vi "ex_ParseFileHeader.vi"(8 "error in (no error)":errorcluster, 11 "file header string":string) -> (0 "error out":errorcluster, 1 "Timestamp":timestamp format="%<%X\n%x>T", 2 "delimiter":string, 3 "file_params":T2={"include col headings?"=TRUE, "x_columns"=0, "col headings always?"=TRUE, "time preference"=0, "hide col headings"=FALSE} {"time preference" items=["Absolute", "Relative"]; "x_columns" items=["None", "One", "Multiple"]}, 4 "optional info":T1, 5 "Decimal Separator":string)   [LabVIEW 2017]
uses:
  <vilib>/express/express input/ExFileReadBlock.llb/ex_ReadFileParams.ctl
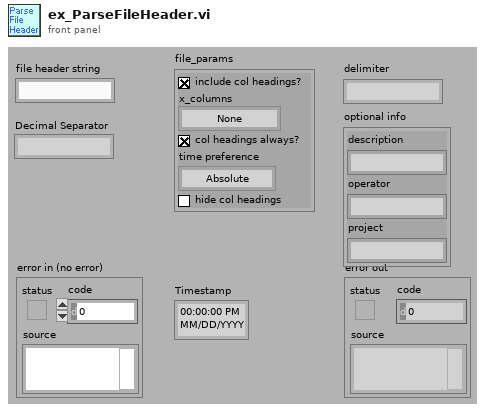
[diagram p1: front panel]
types:
  T1 = cluster{"description":string, "operator":string, "project":string}
  T2 = typedef "ex_ReadFileParams.ctl" = cluster{"include col headings?":bool, "x_columns":u16, "col headings always?":bool, "time preference":u16, "hide col headings":bool}
  T3 = cluster{"Date?":bool, "Time?":bool, "WriterVer?":bool, "ReaderVer?":bool}
  T4 = cluster{"Date":string, "Time":string, "WriterVer":string, "ReaderVer":string}
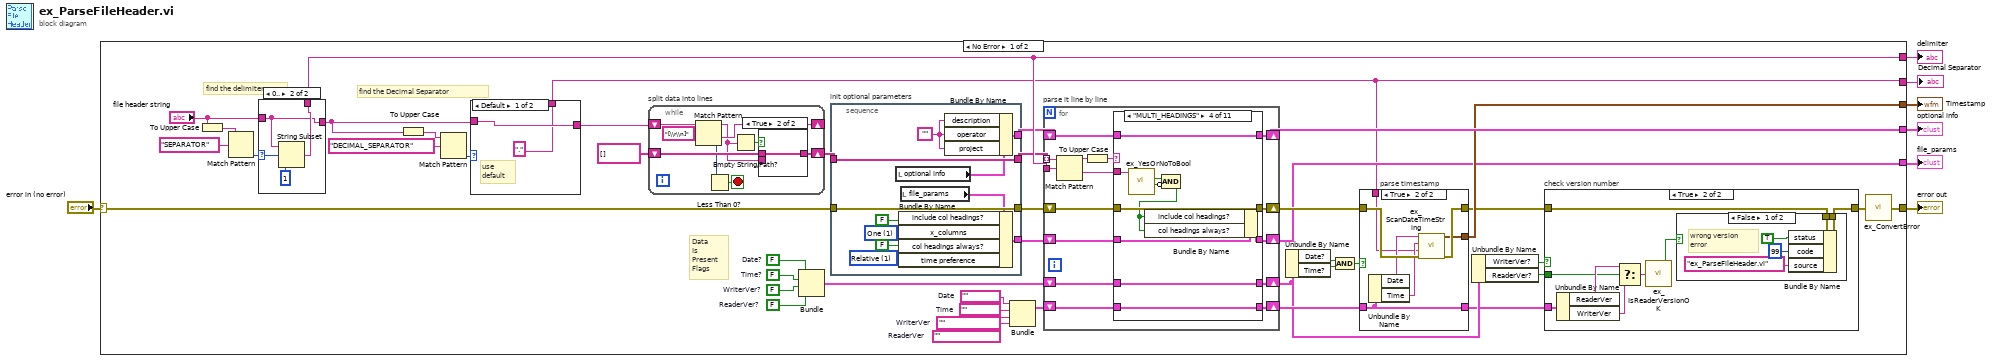
[diagram p0: block diagram]
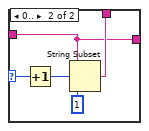
[diagram p2: hidden frame]
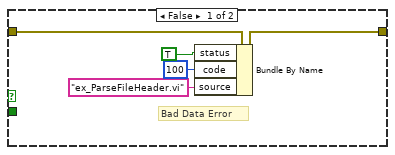
[diagram p3: hidden frame]
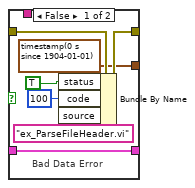
[diagram p5: hidden frame]
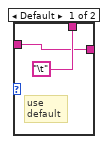
[diagram p6: hidden frame]
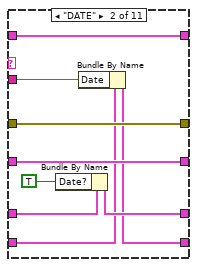
[diagram p8: hidden frame]
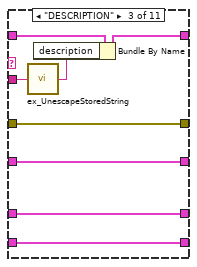
[diagram p9: hidden frame]
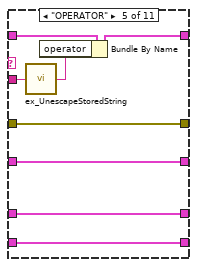
[diagram p10: hidden frame]
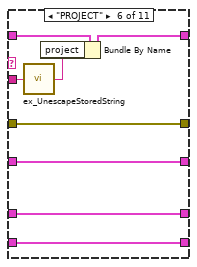
[diagram p11: hidden frame]
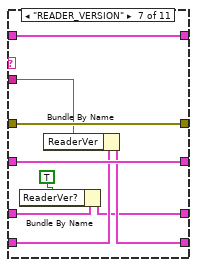
[diagram p12: hidden frame]
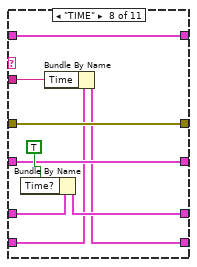
[diagram p13: hidden frame]
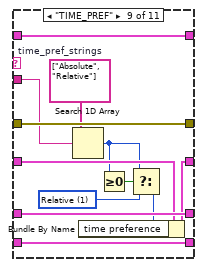
[diagram p14: hidden frame]
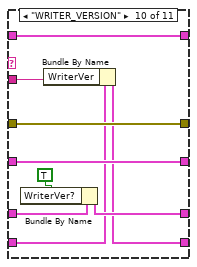
[diagram p15: hidden frame]
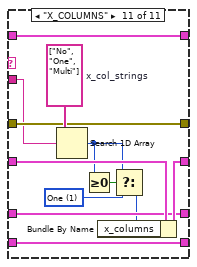
[diagram p16: hidden frame]
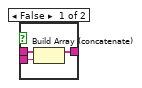
[diagram p17: hidden frame]
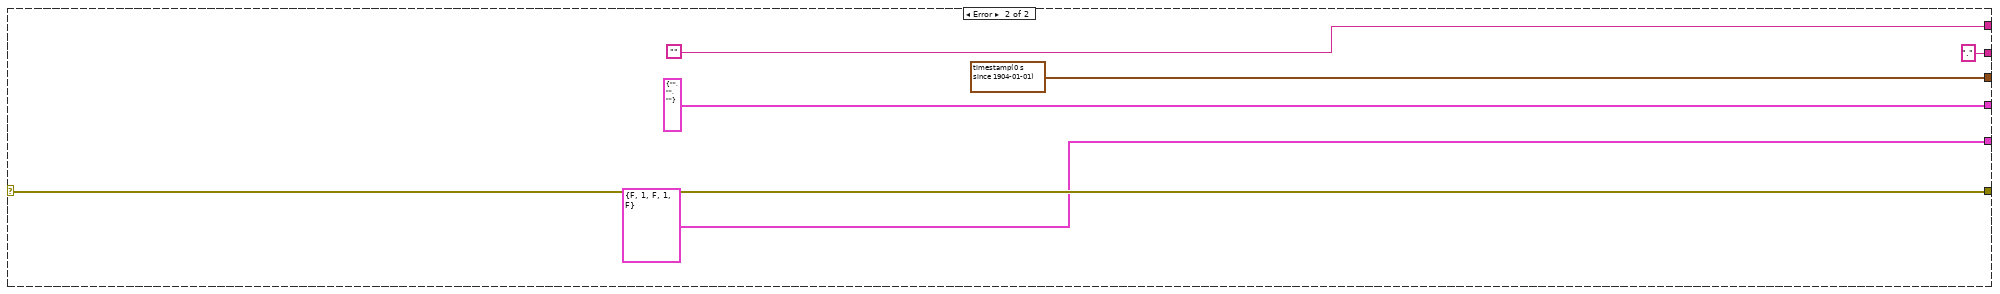
[diagram p18: hidden frame]
diagram:
  n1 = case shown="No Error" "error in (no error)" {
    selector: "error in (no error)" -> [w38 w240]
    tunnel: [w16 w240] -> w6
    tunnel: [w49 ""] -> w5
    tunnel: [w35 T1 {"description"="", "operator"="", "project"=""} ("optional info")] -> w3
    tunnel: [w17 T2 {"include col headings?"=FALSE, "x_columns"=1, "col headings always?"=FALSE, "time preference"=1, "hide col headings"=FALSE} ("file_params")] -> w4
    tunnel: [w23 timestamp(0 s since 1904-01-01)] -> w2
    tunnel: [w8 "." ("file header string")] -> w1
    frame No Error {
      w31 = ""  # ReaderVer
      w30 = ""  # WriterVer
      w32 = FALSE  # ReaderVer?
      w29 = ""  # Time
      w34 = ""  # Date
      w43 = FALSE  # WriterVer?
      w45 = FALSE  # Time?
      w44 = FALSE  # Date?
      # "find the Decimal Separator"
      # "Data\nIs\nPresent\nFlags"
      # "find the delimiter"
      n2 = To Upper Case(1:"file header string") -> (0:w12:string)
      n3 = Match Pattern(string=w12, regular expression="SEPARATOR") -> (offset past match=w47:i32)  [unwired: 4 out]
      n4 = case shown="0.." w47 {
        selector: w47 -> [_ w105]
        tunnel: "file header string" -> [w102 w104]
        tunnel: ["\t" w107] -> w49
        tunnel: [w102 w104] -> w10
        frame Default {
          # "use\ndefault"
        }
        frame 0.. {
          n5 = String Subset(string=w104, offset (0)=w105, length (rest)=1 ("length (rest)")) -> (substring=w107:string)
        }
      }
      n6 = To Upper Case(1:w10) -> (0:w9:string)
      n7 = Match Pattern(string=w9, regular expression="DECIMAL_SEPARATOR") -> (offset past match=w13:i32)  [unwired: 4 out]
      n8 = case shown="Default" w13 {
        selector: w13 -> [_ w54]
        tunnel: w10 -> [w52 w55]
        tunnel: ["." w57] -> w8
        tunnel: [w52 w55] -> w11
        frame Default {
          # "use\ndefault"
        }
        frame 0.. {
          n9 = Increment(x=w54) -> (x+1=w53:i32)
          n10 = String Subset(string=w55, offset (0)=w53, length (rest)=1 ("length (rest)")) -> (substring=w57:string)
        }
      }
      n11 = while "split data into lines" {
        shift-right: [w224] -> _
        shift-left: w11 -> [w230]
        shift-right: [w228] -> w41
        shift-left: string[] [] -> [w229]
        stop <- w226 stop-if-true
        n12 = Match Pattern(string=w230, regular expression="[\\r\\n]") -> (before substring=w223:string, after substring=w224:string, offset past match=w227:i32)  [unwired: 2 out]
        n13 = Less Than 0?(x=w227) -> (x < 0?=w226:bool)
        n14 = Empty String/Path?(string/path=w223) -> (empty?=w222:bool)
        n15 = case shown="True" w222 {
          tunnel: w229 -> [w233 w234]
          tunnel: w223 -> [w232 _]
          tunnel: [w231 w234] -> w228
          frame False {
            n16 = Build Array (concatenate)(w233, w232) -> (w231:string[])
          }
          frame True {
          }
        }
      }
      n17 = Bundle("Date?"=w44, "Time?"=w45, "WriterVer?"=w43, "ReaderVer?"=w32) -> (w42:T3)  [unwired: 1 out]
      n18 = stacked-sequence "init optional parameters" {
        tunnel: w41 -> [w101]
        tunnel: [w101] -> w40
        tunnel: [w100] -> w39
        tunnel: w38 -> [w100]
        tunnel: [w94] -> w37
        tunnel: [w92] -> w36
        frame #0 {
          w91 = ""
          w95 = u16 1 items=["Absolute", "Relative"] ("time preference")
          w97 = u16 1 items=["None", "One", "Multiple"] ("x_columns")
          n19 = local read "optional info"() -> (w93:T1)
          n20 = local read "file_params"() -> (w99:T2)
          n21 = Bundle By Name(cluster=w99, "include col headings?"=FALSE, "x_columns"=w97, "col headings always?"=FALSE, "time preference"=w95) -> (w94:T2)
          n22 = Bundle By Name(cluster=w93, "description"=w91, "operator"=w91, "project"=w91) -> (w92:T1)
        }
      }
      n23 = Bundle("Date"=w34, "Time"=w29, "WriterVer"=w30, "ReaderVer"=w31) -> (w33:T4)  [unwired: 1 out]
      n24 = for "parse it line by line" {
        tunnel: w40 -> [w122] mode=indexing
        tunnel: w49 -> [w121]
        shift-right: [w116] -> w26
        shift-left: w39 -> [w117]
        shift-right: [w109] -> w22
        shift-left: w42 -> [w111]
        shift-right: [w112] -> w17
        shift-left: w37 -> [w113]
        shift-right: [w114] -> w35
        shift-left: w36 -> [w115]
        shift-right: [w108] -> w24
        shift-left: w33 -> [w110]
        n25 = Match Pattern(string=w122, regular expression=w121) -> (before substring=w120:string, after substring=w118:string)  [unwired: 3 out]
        n26 = To Upper Case(1:w120) -> (0:w119:string)
        n27 = case shown="\"MULTI_HEADINGS\"" w119 {
          tunnel: w118 -> [_ w129 w138 w150 w156 w164 w171 w181 w195 w203 w218]
          tunnel: w117 -> [w127 w135 w142 w153 w160 w168 w177 w184 w199 w208 w220]
          tunnel: [w127 w135 w142 w153 w160 w168 w177 w184 w199 w208 w220] -> w116
          tunnel: w115 -> [w126 w136 w144 w154 w162 w170 w179 w183 w200 w209 w219]
          tunnel: [w126 w136 w143 w154 w161 w169 w179 w183 w200 w209 w219] -> w114
          tunnel: w113 -> [w125 w134 w141 w147 w159 w167 w178 w185 w194 w207 w217]
          tunnel: [w125 w134 w141 w146 w159 w167 w178 w185 w193 w207 w216] -> w112
          tunnel: w111 -> [w124 w133 w140 w152 w158 w166 w174 w188 w198 w206 w215]
          tunnel: w110 -> [w123 w130 w139 w151 w157 w165 w176 w182 w197 w202 w214]
          tunnel: [w124 w131 w140 w152 w158 w166 w173 w187 w198 w205 w215] -> w109
          tunnel: [w123 w128 w139 w151 w157 w165 w175 w180 w197 w201 w214] -> w108
          frame Default {
          }
          frame "DATE" {
            n28 = Bundle By Name(cluster=w133, "Date?"=TRUE) -> (w131:T3)
            n29 = Bundle By Name(cluster=w130, "Date"=w129) -> (w128:T4)
          }
          frame "DESCRIPTION" {
            n30 = call <vilib>:"ex_UnescapeStoredString.vi"("stored string"=w138) -> ("parsed string"=w137:string)
            n31 = Bundle By Name(cluster=w144, "description"=w137) -> (w143:T1)
          }
          frame "MULTI_HEADINGS" {
            n32 = call <vilib>:"ex_YesOrNoToBool.vi"("YesOrNo String"=w150) -> ("error"=w148:bool, "Yes?"=w149:bool)  [unwired: 8 out]
            n33 = Compound Arithmetic op=AND(w149, invert w148) -> (w145:bool)
            n34 = Bundle By Name(cluster=w147, "include col headings?"=w145, "col headings always?"=w145) -> (w146:T2)
          }
          frame "OPERATOR" {
            n35 = call <vilib>:"ex_UnescapeStoredString.vi"("stored string"=w156) -> ("parsed string"=w155:string)
            n36 = Bundle By Name(cluster=w162, "operator"=w155) -> (w161:T1)
          }
          frame "PROJECT" {
            n37 = call <vilib>:"ex_UnescapeStoredString.vi"("stored string"=w164) -> ("parsed string"=w163:string)
            n38 = Bundle By Name(cluster=w170, "project"=w163) -> (w169:T1)
          }
          frame "READER_VERSION" {
            n39 = Bundle By Name(cluster=w174, "ReaderVer?"=TRUE) -> (w173:T3)
            n40 = Bundle By Name(cluster=w176, "ReaderVer"=w171) -> (w175:T4)
          }
          frame "TIME" {
            n41 = Bundle By Name(cluster=w188, "Time?"=TRUE) -> (w187:T3)
            n42 = Bundle By Name(cluster=w182, "Time"=w181) -> (w180:T4)
          }
          frame "TIME_PREF" {
            w196 = string[] ["Absolute", "Relative"]  # time_pref_strings
            w189 = u16 1 items=["Absolute", "Relative"] ("time preference")
            n43 = Search 1D Array(1D array=w196, element=w195) -> (index of element=w191:i32)  [unwired: 1 out]
            n44 = Greater Or Equal To 0?(x=w191) -> (x >= 0?=w192:bool)
            n45 = Select(t=w191, s=w192, f=w189) -> (s? t:f=w190:i32)
            n46 = Bundle By Name(cluster=w194, "time preference"=w190) -> (w193:T2)
          }
          frame "WRITER_VERSION" {
            n47 = Bundle By Name(cluster=w206, "WriterVer?"=TRUE) -> (w205:T3)
            n48 = Bundle By Name(cluster=w202, "WriterVer"=w203) -> (w201:T4)
          }
          frame "X_COLUMNS" {
            w221 = string[] ["No", "One", "Multi"]  # x_col_strings
            w212 = u16 1 items=["None", "One", "Multiple"] ("x_columns")
            n49 = Search 1D Array(1D array=w221, element=w218) -> (index of element=w210:i32)  [unwired: 1 out]
            n50 = Greater Or Equal To 0?(x=w210) -> (x >= 0?=w211:bool)
            n51 = Select(t=w210, s=w211, f=w212) -> (s? t:f=w213:i32)
            n52 = Bundle By Name(cluster=w217, "x_columns"=w213) -> (w216:T2)
          }
        }
      }
      n53 = Unbundle By Name(w22) -> ("Date?"=w27:bool, "Time?"=w28:bool)
      n54 = And(x=w27, y=w28) -> (x .and. y?=w25:bool)
      n55 = case "parse timestamp" shown="True" w25 {
        tunnel: w26 -> [w80 w90]
        tunnel: w24 -> [w77 w86]
        tunnel: [w79 w87] -> w20
        tunnel: [timestamp(0 s since 1904-01-01) w85] -> w23
        tunnel: [w77 w86] -> w18
        tunnel: w8 -> [_ w84]
        frame False {
          # "Bad Data Error"
          n56 = Bundle By Name(cluster=w80, "status"=TRUE, "code"=100, "source"="ex_ParseFileHeader.vi") -> (w79:errorcluster)
        }
        frame True {
          n57 = Unbundle By Name(w86) -> ("Date"=w89:string, "Time"=w88:string)
          n58 = call <vilib>:"ex_ScanDateTimeString.vi"("error in (no error)"=w90, "Decimal point"=w84, "Time String"=w88, "Date String"=w89) -> ("error out"=w87:errorcluster, "Date/Time in seconds"=w85:timestamp)  [unwired: 2 out]
        }
      }
      n59 = Unbundle By Name(w22) -> ("WriterVer?"=w21:bool, "ReaderVer?"=w19:bool)
      n60 = case "check version number" shown="True" w21 {
        tunnel: w20 -> [w59 w64]
        tunnel: [w58 w63] -> w15
        tunnel: w19 -> [_ w68]
        tunnel: w18 -> [_ w70]
        frame False {
          # "Bad Data Error"
          n61 = Bundle By Name(cluster=w59, "status"=TRUE, "code"=100, "source"="ex_ParseFileHeader.vi") -> (w58:errorcluster)
        }
        frame True {
          n62 = Unbundle By Name(w70) -> ("ReaderVer"=w69:string, "WriterVer"=w67:string)
          n63 = Select(t=w69, s=w68, f=w67) -> (s? t:f=w66:string)
          n64 = call <vilib>:"ex_IsReaderVersionOK.vi"("Reader Version"=w66) -> ("OK?"=w65:bool)
          n65 = case shown="False" w65 {
            tunnel: w64 -> [w74 w76]
            tunnel: [w73 w76] -> w63
            frame False {
              # "wrong version\nerror"
              n66 = Bundle By Name(cluster=w74, "status"=TRUE, "code"=99, "source"="ex_ParseFileHeader.vi") -> (w73:errorcluster)
            }
            frame True {
            }
          }
        }
      }
      n67 = call <vilib>:"ex_ConvertError.vi"("error in (no error)"=w15) -> ("error out"=w16:errorcluster)  [unwired: 4 out]
    }
    frame Error {
    }
  }
  "file_params" <- w4
  "error out" <- w6
  "delimiter" <- w5
  "Timestamp" <- w2
  "optional info" <- w3
  "Decimal Separator" <- w1
